vi "FTW-Reply-Listener.vi"(1 "Endpoint":refnum<class "FTW-Endpoint.lvclass">, 2 "Message Handler":refnum<user-event>) -> ()   [LabVIEW 2013, in "FTW-Reply.lvclass"]
uses:
  FTW-Reply.lvclass
  Message/Request/FTW-Message-IncomingRequest.lvclass
  Endpoint/FTW-Endpoint.lvclass
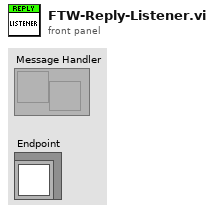
[diagram p1: front panel]
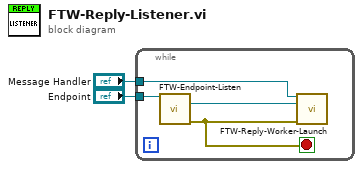
[diagram p0: block diagram]
diagram:
  n1 = while {
    tunnel: "Message Handler" -> [w5]
    tunnel: "Endpoint" -> [w6]
    stop <- w4 stop-if-true
    n2 = call-dynamic "FTW-Endpoint-Listen.vi"("FTW Endpoint"=w6) -> ("New Connection"=w3:refnum<class "FTW-Endpoint.lvclass">, "error out"=w4:errorcluster)  [unwired: 12 in, 1 out]
    n3 = call "FTW-Reply-Worker-Launch.vi"("Message Handler"=w5, "FTW-Endpoint in"=w3, "error in"=w4) -> ()  [unwired: 12 in, 1 out]
  }
